vi "K6221_GetSetPoint.vi"(8 "port":u16=3375, 9 "Data mac ip address":string="146.201.201.70", 11 "VISA resource name":refnum<visa-resource-name>="GPIB0::20::INSTR") -> (0 "Current Set Point (mA)":dbl=-17.9883723 format="%#_4g", 3 "VISA resource name Out":refnum<visa-resource-name>="GPIB0::20::INSTR")   [LabVIEW 2018]
panel:
  out "error out":errorcluster
  in  "error in (no error)":errorcluster
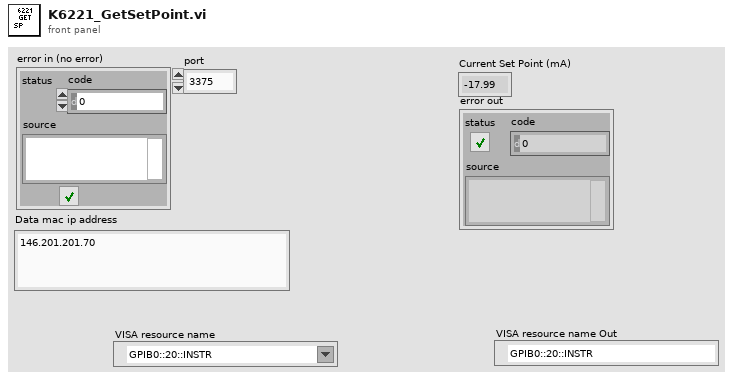
[diagram p1: front panel]
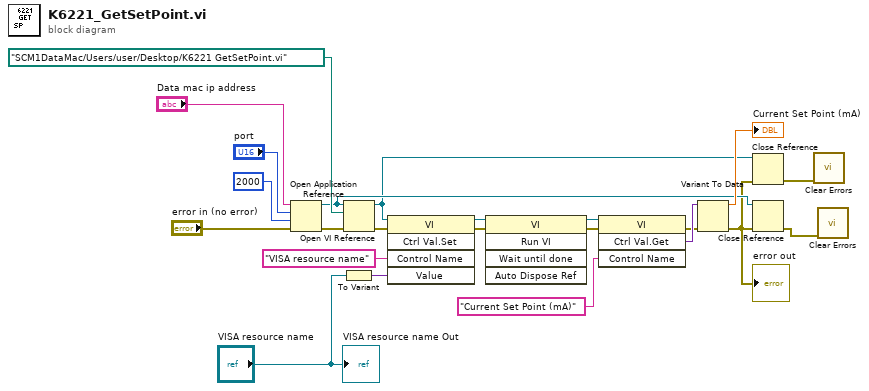
[diagram p0: block diagram]
diagram:
  n1 = Open Application Reference(8:"error in (no error)", 9:2000 ("timeout ms (60000)"), 10:"port", 11:"Data mac ip address") -> (0:w4:errorcluster, 3:w7:refnum<vi>)
  n2 = Open VI Reference(application reference (local)=w7, vi path=path "/SCM1DataMac/Users/user/Desktop/K6221 GetSetPoint.vi", error in (no error)=w4) -> (vi reference=w6:refnum<vi>, error out=w5:errorcluster)  [unwired: 3 in]
  n3 = To Variant(anything="VISA resource name") -> (Variant=w9:variant)
  n4 = invoke class="VI" method="Ctrl Val.Set"(reference=w6, error in=w5, "Control Name"="VISA resource name", "Value"=w9) -> (reference out=w12:refnum<vi>, error out=w11:errorcluster)  [unwired: 1 in, 3 out]
  n5 = invoke class="VI" method="Run VI"(reference=w12, error in=w11) -> (reference out=w15:refnum<vi>, error out=w14:errorcluster)  [unwired: 3 in, 3 out]
  n6 = invoke class="VI" method="Ctrl Val.Get"(reference=w15, error in=w14, "Control Name"="Current Set Point (mA)") -> (error out=w17:errorcluster, "Get Control Value Variant"=w18:variant)  [unwired: 1 in, 2 out]
  n7 = Variant To Data(error in=w17, Variant=w18) -> (data=→"Current Set Point (mA)":dbl, error out=w3:errorcluster)  [unwired: 1 in]
  "error out" <- w3
  n8 = Close Reference(reference=w6, error in (no error)=w3) -> (error out=w2:errorcluster)
  n9 = Close Reference(reference=w7, error in (no error)=w3) -> (error out=w1:errorcluster)
  n10 = call <vilib>:"Clear Errors.vi"("error in (no error)"=w2) -> ()  [unwired: 5 in, 2 out]
  n11 = call <vilib>:"Clear Errors.vi"("error in (no error)"=w1) -> ()  [unwired: 5 in, 2 out]
  "VISA resource name Out" <- "VISA resource name"
